vi "Save Tree Collapsed State.vi"(11 "Message Maker in":refnum<class "Message Maker.lvclass">) -> (1 "Array":string[](array[string]), 3 "Message Maker out":refnum<class "Message Maker.lvclass">)   [LabVIEW 2023, in "Message Maker.lvclass"]
uses:
  Message Maker.lvclass
  Message Maker.lvclass/Message Maker.ctl
panel:
  out "Actors Tree ref":refnum<vi>
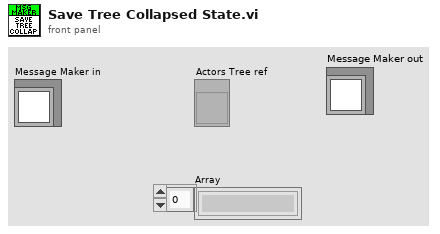
[diagram p1: front panel]
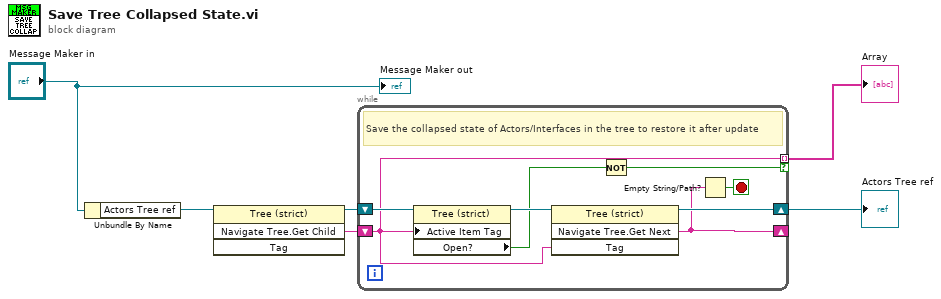
[diagram p0: block diagram]
diagram:
  n1 = Unbundle By Name("Message Maker in") -> ("Actors Tree ref"=w2:refnum<vi>)
  n2 = invoke class="Tree (strict)" method="Navigate Tree.Get Child"(reference=w2) -> (reference out=w3:refnum<vi>, "Navigate Tree:Get Child"=w4:string)  [unwired: 3 in, 2 out]
  n3 = while {
    shift-right: [w11] -> _
    shift-left: w4 -> [w8]
    shift-right: [w12] -> w5
    shift-left: w3 -> [w14]
    tunnel: [w8] -> w6 mode=indexing if=w7
    stop <- w10 stop-if-true
    # "Save the collapsed state of Actors/Interfaces in the tree to restore it after update"
    n4 = property class="Tree (strict)"(reference=w14, "Active Item Tag"=w8) -> (reference out=w13:refnum<vi>, "Open?"=w9:bool)  [unwired: 1 in, 1 out]
    n5 = invoke class="Tree (strict)" method="Navigate Tree.Get Next"(reference=w13, "Tag"=w8) -> (reference out=w12:refnum<vi>, "Navigate Tree:Get Next Item"=w11:string)  [unwired: 2 in, 2 out]
    n6 = Not(x=w9) -> (.not. x?=w7:bool)
    n7 = Empty String/Path?(string/path=w11) -> (empty?=w10:bool)
  }
  "Array" <- w6
  "Actors Tree ref" <- w5
  "Message Maker out" <- "Message Maker in"
